vi "Write Legend Minimum.vi"(5 "Legend Minimum":u32, 9 "WaveformChart in":refnum<class "WaveformChart.lvclass">) -> (3 "WaveformChart out":refnum<class "WaveformChart.lvclass">)   [LabVIEW 2014, in "Raspberry Pi Compatible Compiler for LabVIEW.lvlib" / "WaveformChart.lvclass"]
uses:
  WaveformChart.lvclass
  WaveformChart.lvclass/WaveformChart.ctl
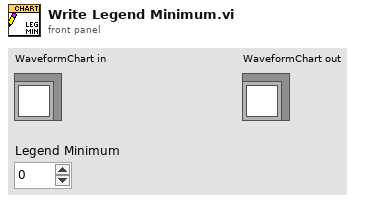
[diagram p1: front panel]
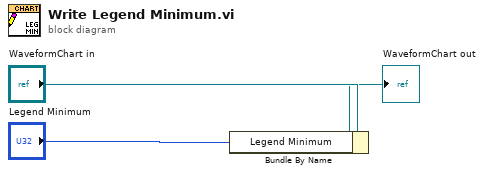
[diagram p0: block diagram]
diagram:
  n1 = Bundle By Name(cluster="WaveformChart in", "Legend Minimum"="Legend Minimum") -> (→"WaveformChart out":refnum<class "WaveformChart.lvclass">)
